vi "IRselection pulse nettoyé_SD.vi"(1 "DATA":dbl[](array[numeric])=array[55296 elements]) -> (0 "résultat pulse nettoyé":dbl[](array[numeric]))   [LabVIEW 2015]
uses:
  globalVarSD.vi
panel:
  out "Data":dbl[](graph)
  out "Res":dbl[](graph)
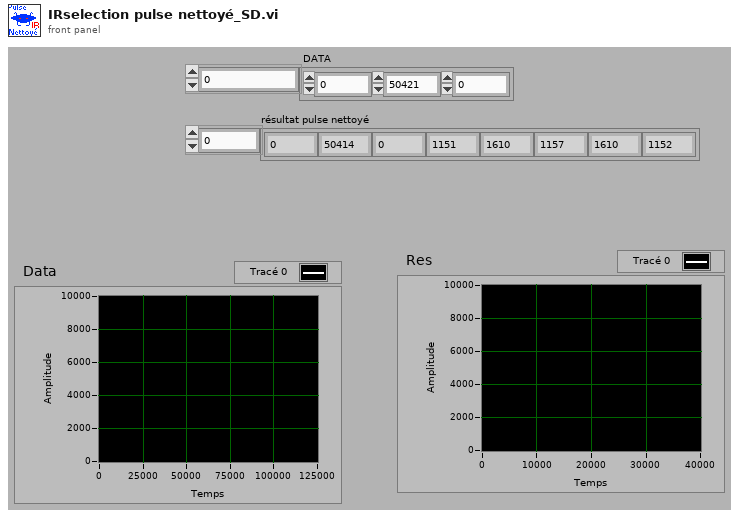
[diagram p1: front panel]
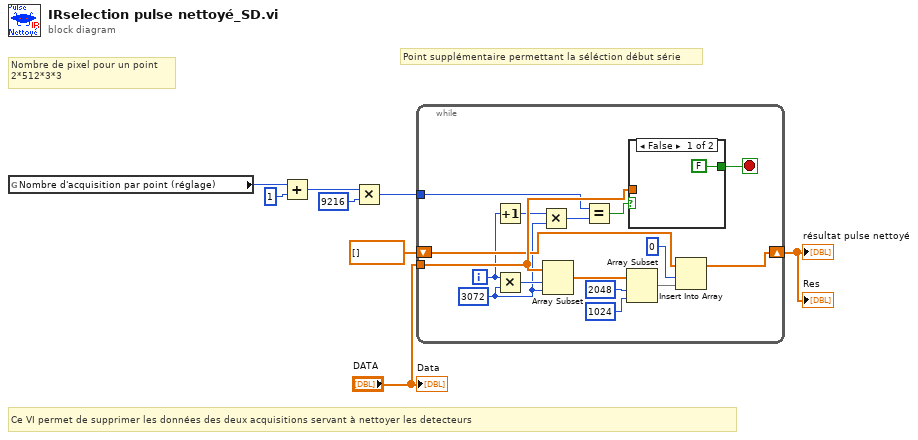
[diagram p0: block diagram]
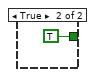
[diagram p2: hidden frame]
diagram:
  # "Nombre de pixel pour un point\n2*512*3*3"
  # "Ce VI permet de supprimer les données des deux acquisitions servant à nettoyer les detecteurs"
  # "Point supplémentaire permettant la séléction début série"
  n1 = global read "globalVarSD.vi" "Nombre d'acquisition par point (réglage)"() -> (w3:u32)
  n2 = Add(x=w3, y=1) -> (x+y=w8:u32)
  n3 = Multiply(x=w8, y=9216) -> (x*y=w5:u32)
  n4 = while {
    tunnel: "DATA" -> [w22]
    tunnel: w5 -> [w14]
    shift-right: [w17] -> w1
    shift-left: dbl[] [] -> [w16]
    i -> [w13]
    stop <- w24 stop-if-true
    w11 = 3072 ("x")
    n5 = Increment(x=w13) -> (x+1=w12:i32)
    n6 = Multiply(x=w13, y=w11) -> (x*y=w23:i32)
    n7 = Multiply(x=w12, y=w11) -> (x*y=w10:i32)
    n8 = Array Subset(array=w22, index=w23, length=w11) -> (w21:dbl[])
    n9 = Equal?(x=w14, y=w10) -> (x = y?=w9:bool)
    n10 = Array Subset(array=w21, index=2048 ("indice"), length=1024 ("longueur")) -> (w18:dbl[])
    n11 = case shown="False" w9 {
      tunnel: w22 -> [_ _]
      tunnel: [FALSE TRUE] -> w24
      frame False {
      }
      frame True {
      }
    }
    n12 = Insert Into Array(array=w16, index=0 ("indice"), new element=w18) -> (w17:dbl[])
  }
  "résultat pulse nettoyé" <- w1
  "Res" <- w1
  "Data" <- "DATA"
